vi "download_calibration_rm_depth_longthrow.vi"(9 "port":u16, 10 "host":string, 11 "path in":path=path "hl2ss_ulm.dll") -> (1 "error":bool, 2 "calibration":T1, 3 "path out":path)   [LabVIEW 2023]
panel:
  in  "calibration":T1
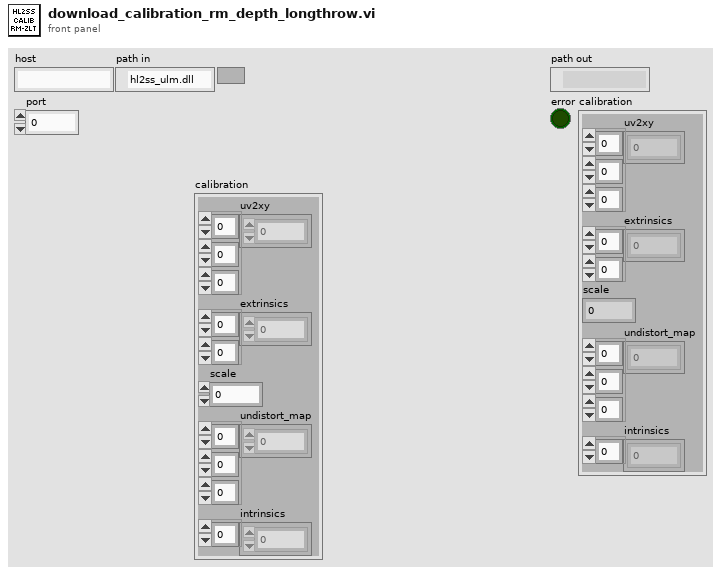
[diagram p1: front panel]
types:
  T1 = cluster{"uv2xy":sgl[][][], "extrinsics":sgl[][], "scale":sgl, "undistort_map":sgl[][][], "intrinsics":sgl[]}
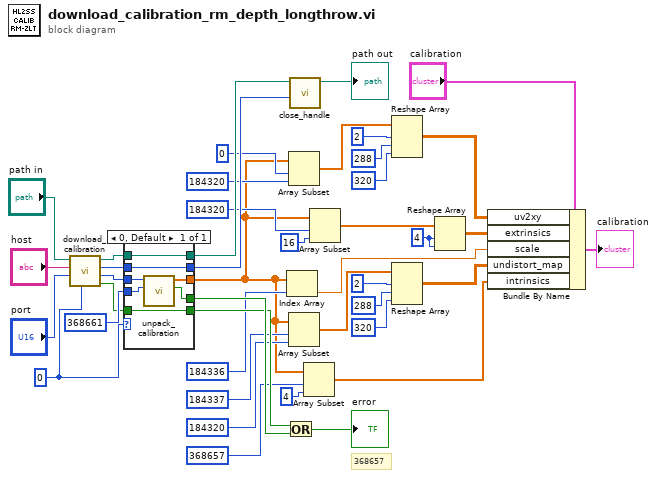
[diagram p0: block diagram]
diagram:
  w9 = 4 ("dimension size")
  w39 = u64 0 ("configuration")
  # "368657"
  n1 = call "download_calibration.vi"("configuration"=w39, "port"="port", "host"="host", "path in"="path in") -> ("error"=w28:bool, "calibration"=w37:u64, "calibration_handle"=w35:u64, "path out"=w36:path)  [unwired: 4 in]
  n2 = case shown="0, Default" w39 {
    tunnel: 368661 ("element_count") -> [w49]
    tunnel: w37 -> [w48]
    tunnel: w36 -> [w47]
    tunnel: w35 -> [w46]
    tunnel: [w47] -> w34
    tunnel: [w46] -> w33
    tunnel: [w45] -> w18
    tunnel: [w44] -> w32
    tunnel: [w43] -> w29
    tunnel: w28 -> [w43]
    frame 0, Default {
      n3 = call "unpack_calibration.vi"("element_count"=w49, "calibration"=w48) -> ("error"=w44:bool, "calibration"=w45:sgl[])  [unwired: 8 in]
    }
  }
  n4 = Or(x=w29, y=w32) -> (x .or. y?=→"error":bool)
  n5 = Index Array(array=w18, index=184336) -> (element=w2:sgl)
  n6 = Array Subset(array=w18, index=0, length=184320) -> (w10:sgl[])
  n7 = Array Subset(array=w18, index=184337, length=184320) -> (w17:sgl[])
  n8 = call "close_handle.vi"("handle"=w33, "path in"=w34) -> ("path out"=→"path out":path)  [unwired: 9 in]
  n9 = Array Subset(array=w18, index=368657, length=4) -> (w3:sgl[])
  n10 = Array Subset(array=w18, index=184320, length=16) -> (w8:sgl[])
  n11 = Reshape Array(w10, 2 ("dimension size"), 288 ("dimension size"), 320 ("dimension size")) -> (w1:sgl[][][])
  n12 = Reshape Array(w17, 2 ("dimension size"), 288 ("dimension size"), 320 ("dimension size")) -> (w4:sgl[][][])
  n13 = Reshape Array(w8, w9, w9) -> (w5:sgl[][])
  n14 = Bundle By Name(cluster="calibration", "uv2xy"=w1, "extrinsics"=w5, "scale"=w2, "undistort_map"=w4, "intrinsics"=w3) -> (→"calibration":T1)
